vi "Initialize.vi"(8 "error in":errorcluster) -> (0 "error out":errorcluster, 3 "CoreOOB_Tx out":refnum<class "CIFCoreOOB_Tx.lvclass">)   [LabVIEW 2021, in "CIFCoreOOB_Tx.lvclass"]
uses:
  CIFCoreOOB_Tx.lvclass
  D:/dev/CIF-LVCore/src/CIFUtilities/CIFOutOfBand/CIFOutOfBand.lvclass
  Typedef/Template Payload.ctl
  Common/Typedef/Plugin Status.ctl
  Common/Typedef/Plugin State.ctl
  Common/Typedef/Timing Statistics.ctl
  Common/Typedef/Timing Stats Base.ctl
  Common/Typedef/FIFO Statistics.ctl
  Common/Typedef/Simple Error.ctl
  Common/Typedef/Monitor Doubles.ctl
  Common/Typedef/Monitor U64.ctl
  Common/Typedef/Monitor I64.ctl
  Common/Typedef/Plugin Overrides.ctl
  Common/Typedef/Timing Overrides.ctl
  Channels/CIFChannelMng/typedef/Channel List for OOB.ctl
  Channels/CIFChannels/Typedef/Direction.ctl
  CIFUtilities/CIFOutOfBand/CIFOutOfBand.lvclass/CIFOutOfBand.ctl
  CIFUtilities/CIFOutOfBand/CIFOutOfBand.lvclass
  Common/CIFCoreCommon.lvlib
  Channels/CIFChannels/CIFChannels.lvclass
  Channels/CIFChannelMng/CIFChannelMng.lvclass
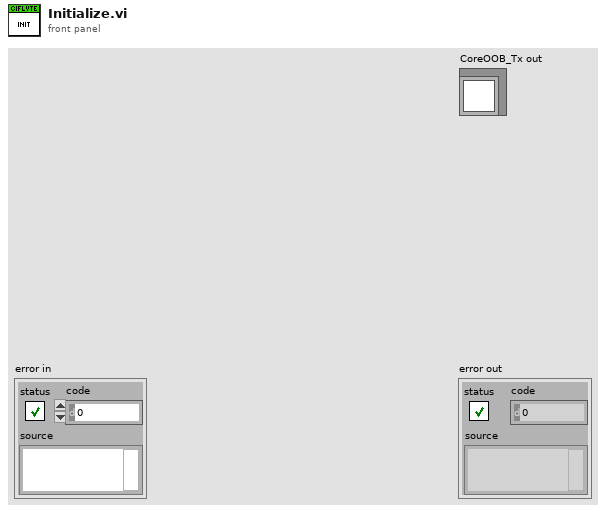
[diagram p1: front panel]
types:
  T1 = typedef "CIFCoreOOB_Tx.lvclass/Template Payload.ctl" = cluster{"Status":T2, "Plugin Overrides":T11, "Channel List":T13[]}
  T2 = typedef "CIFCoreCommon.lvlib/Plugin Status.ctl" = cluster{"State":T3, "Timing Statistics (us)":T4, "FIFO Statistics (us)":T6, "error":T7, "Monitor Doubles":T8, "Monitor U64":T9, "Monitor I64":T10, "Cleanup":T5, "Create":i32, "Destroy":i32}
  T3 = typedef "CIFCoreCommon.lvlib/Plugin State.ctl" = enum32{"Null", "Creating", "Listening", "Running", "CleaningUp", "Destroying"}
  T4 = typedef "CIFCoreCommon.lvlib/Timing Statistics.ctl" = cluster{"Period":T5, "Wake Error":T5, "Execute":T5, "Housekeep":T5, "Idle":T5}
  T5 = typedef "CIFCoreCommon.lvlib/Timing Stats Base.ctl" = cluster{"Max":i32, "Min":i32}
  T6 = typedef "CIFCoreCommon.lvlib/FIFO Statistics.ctl" = cluster{"From T0":T5, "From Previous Plugin":T5, "Output Error":T5}
  T7 = typedef "CIFCoreCommon.lvlib/Simple Error.ctl" = cluster{"status":bool, "code":i32}
  T8 = typedef "CIFCoreCommon.lvlib/Monitor Doubles.ctl" = cluster{"1":dbl, "2":dbl, "3":dbl, "4":dbl}
  T9 = typedef "CIFCoreCommon.lvlib/Monitor U64.ctl" = cluster{"1":u64, "2":u64, "3":u64, "4":u64}
  T10 = typedef "CIFCoreCommon.lvlib/Monitor I64.ctl" = cluster{"1":i64, "2":i64, "3":i64, "4":i64}
  T11 = typedef "CIFCoreCommon.lvlib/Plugin Overrides.ctl" = cluster{"Timing Overrides":T12}
  T12 = typedef "CIFCoreCommon.lvlib/Timing Overrides.ctl" = cluster{"Override Timing":bool, "Skip Sleep":bool, "Period (s)":dbl}
  T13 = typedef "CIFChannelMng.lvclass/Channel List for OOB.ctl" = cluster{"Name":string, "Direction":T14, "Type":string, "Connected?":bool, "Connected Name":string, "Custom Config Data":u8[]}
  T14 = typedef "CIFChannels.lvclass/Direction.ctl" = enum16{"Publisher", "Subscriber"}
  T15 = typedef "CIFCoreOOB_Tx.lvclass/OOB Core Commands.ctl" = enum8{"Status", "Overrides", "Channel List"}
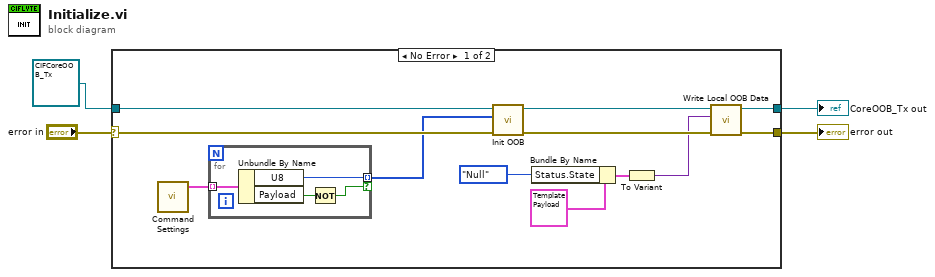
[diagram p0: block diagram]
diagram:
  n1 = case shown="No Error" "error in" {
    selector: "error in" -> [w16 w22]
    tunnel: [w10 w22] -> w3
    tunnel: [w9 w21] -> w2
    tunnel: refnum<class "CIFCoreOOB_Tx.lvclass"> refnum ("CifLvTemplateOutOfBand in") -> [w15 w21]
    frame No Error {
      n2 = call "Command Settings.vi"() -> ("Command Stats"=w14:cluster{"Enum":T15, "U8":u8, "Payload":bool}[])  [unwired: 5 in]
      n3 = for {
        tunnel: w14 -> [w20] mode=indexing
        tunnel: [w19] -> w13 mode=indexing if=w17
        n4 = Unbundle By Name(w20) -> ("U8"=w19:u8, "Payload"=w18:bool)
        n5 = Not(x=w18) -> (.not. x?=w17:bool)
      }
      n6 = call "Init OOB.vi"("error in (no error)"=w16, "Cases to Skip Payload"=w13, "OOB in"=w15) -> ("error out"=w11:errorcluster, "OOB out"=w12:refnum<class "CIFCoreOOB_Tx.lvclass">)  [unwired: 7 in]
      n7 = Bundle By Name(cluster=T1 {"Status"={"State"=enum."Null", "Timing Statistics (us)"={"Period"={"Max"=0, "Min"=0}, "Wake Error"={"Max"=0, "Min"=0}, "Execute"={"Max"=0, "Min"=0}, "Housekeep"={"Max"=0, "Min"=0}, "Idle"={"Max"=0, "Min"=0}}, "FIFO Statistics (us)"={"From T0"={"Max"=0, "Min"=0}, "From Previous Plugin"={"Max"=0, "Min"=0}, "Output Error"={"Max"=0, "Min"=0}}, "error"={"status"=FALSE, "code"=0}, "Monitor Doubles"={"1"=0.0, "2"=0.0, "3"=0.0, "4"=0.0}, "Monitor U64"={"1"=0, "2"=0, "3"=0, "4"=0}, "Monitor I64"={"1"=0, "2"=0, "3"=0, "4"=0}, "Cleanup"={"Max"=0, "Min"=0}, "Create"=0, "Destroy"=0}, "Plugin Overrides"={"Timing Overrides"={"Override Timing"=FALSE, "Skip Sleep"=FALSE, "Period (s)"=0.0}}, "Channel List"=[]} ("Template Payload"), "Status.State"=Plugin_State."Null") -> (w8:T1)
      n8 = To Variant(anything=w8) -> (Variant=w7:variant)
      n9 = call "Write Local OOB Data.vi"("error in"=w11, "Local OOB Data"=w7, "OOB in"=w12) -> ("error out"=w10:errorcluster, "OOB out"=w9:refnum<class "CIFCoreOOB_Tx.lvclass">)  [unwired: 7 in]
    }
    frame Error {
    }
  }
  "error out" <- w3
  "CoreOOB_Tx out" <- w2
